vi "port_facade.vi"(0 "Data In":T4, 2 "Display State In":T2, 3 "Container State":T3) -> (6 "Data Out":T4, 7 "Display State Out":T2, 8 "Action":T1)   [LabVIEW 2024, in "portX.xctl"]
uses:
  Users/crogers/GitHub/ME121-25/LabVIEW/SerialVIs/subs/portX.xctl
  <userlib>/SerialVIs/subs/port_data.ctl
  <vilib>/_xctls/Container State.ctl
  <userlib>/SerialVIs/subs/port_state.ctl
  <vilib>/_xctls/Action.ctl
  <vilib>/_xctls/XControlSupport.lvlib
panel:
  in  "refresh":bool
  in  "Port":u16(ring)
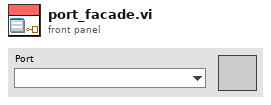
[diagram p1: front panel]
types:
  T1 = typedef "XControlSupport.lvlib/Action.ctl" = cluster{"Data Changed?":bool, "State Changed?":bool, "Action Name":string}
  T2 = typedef "portX.xctl/port_state.ctl" = cluster{"Numeric":dbl}
  T3 = typedef "XControlSupport.lvlib/Container State.ctl" = cluster{"Indicator?":bool, "Run Mode?":bool, " Refnum":refnum<vi>}
  T4 = typedef "portX.xctl/port_data.ctl" = refnum<visa-resource-name>
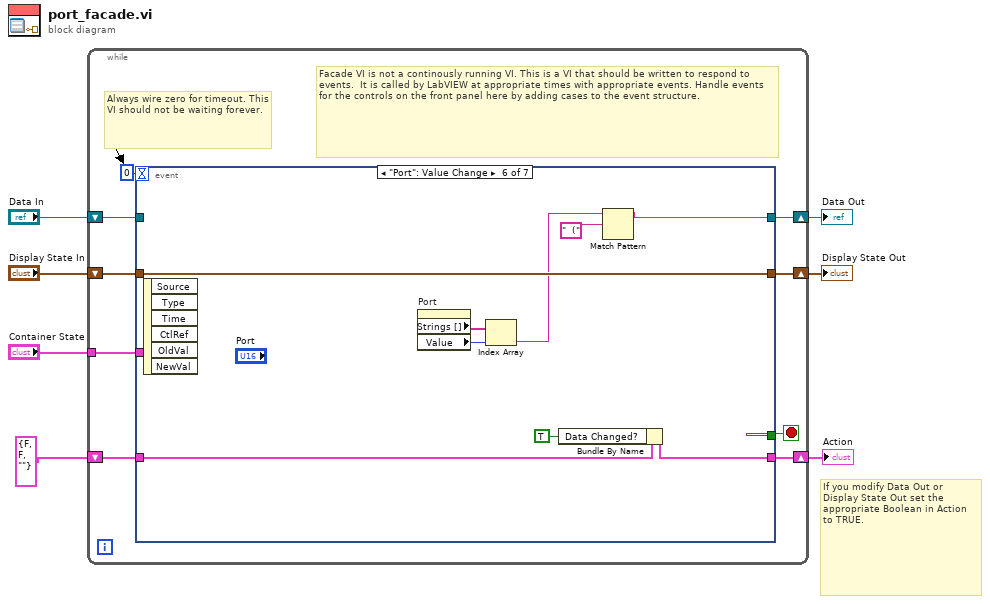
[diagram p0: block diagram]
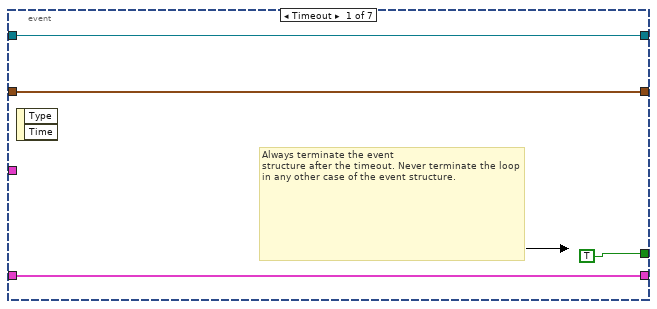
[diagram p2: hidden frame]
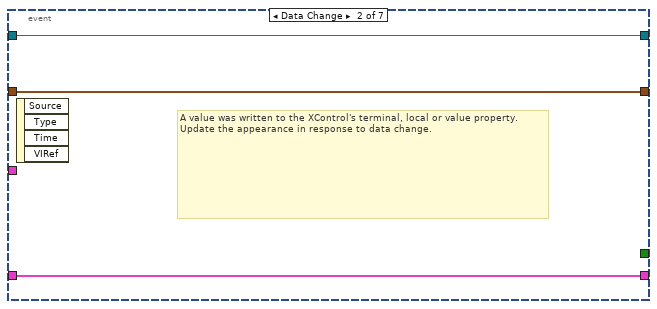
[diagram p3: hidden frame]
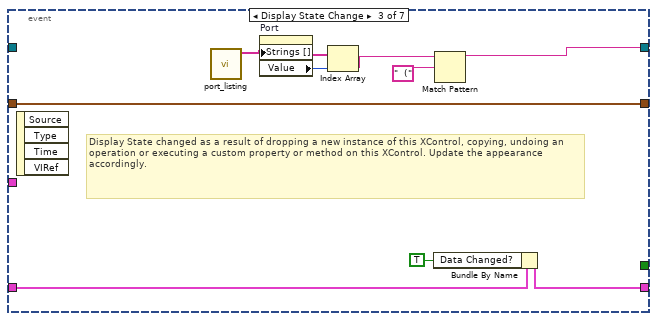
[diagram p4: hidden frame]
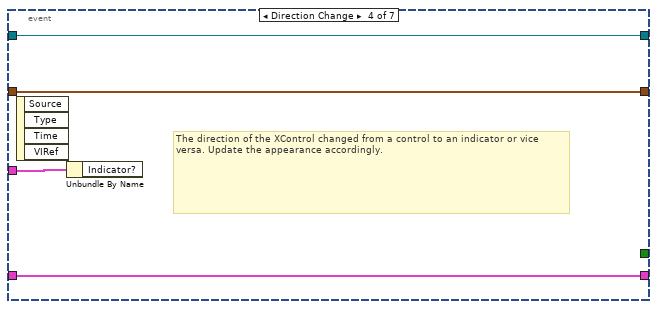
[diagram p5: hidden frame]
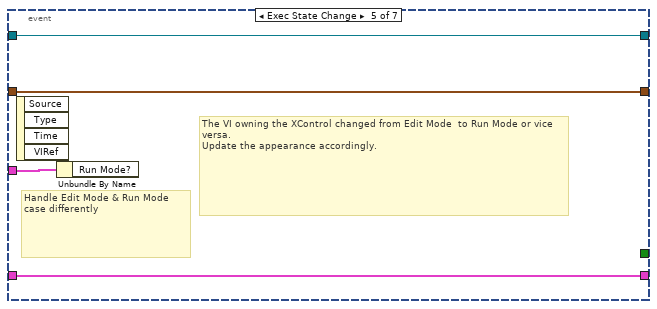
[diagram p6: hidden frame]
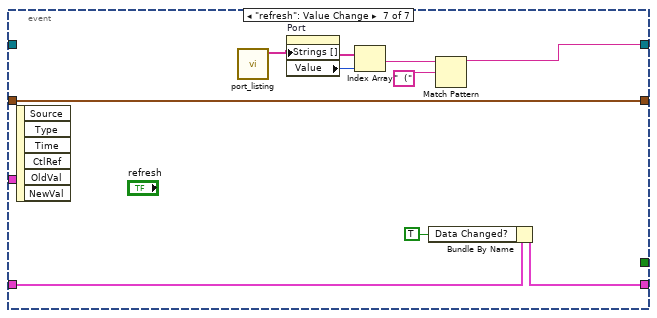
[diagram p7: hidden frame]
diagram:
  # "If you modify Data Out or\nDisplay State Out set the\nappropriate Boolean in Action\nto TRUE."
  n1 = while {
    shift-right: [w15] -> w4
    shift-left: "Display State In" -> [w16]
    tunnel: "Container State" -> [w12]
    shift-right: [w10] -> w7
    shift-left: "Data In" -> [w11]
    shift-right: [w8] -> w2
    shift-left: T1 {"Data Changed?"=FALSE, "State Changed?"=FALSE, "Action Name"=""} ("Action") -> [w9]
    stop <- w14 stop-if-true
    # "Facade VI is not a continously running VI. This is a VI that should be written to respond to events.  It is called by LabVIEW at appropriate times with appropriate events. Handle events for the controls on the front panel here by adding cases to the event structure."
    # "Always wire zero for timeout. This\nVI should not be waiting forever."
    n2 = event shown="[5] \"Port\": Value Change" {
      selector: _ -> [_ _ _ _ _ _ _]
      dyn-events: _ -> [_ _ _ _ _ _ _]
      timeout: 0 -> [_ _ _ _ _ _ _]
      tunnel: w16 -> [w18 w22 w32 w35 w39 w49 w58]
      tunnel: [w18 w22 w32 w35 w39 w49 w58] -> w15
      tunnel: [TRUE _ _ _ _ _ _] -> w14
      tunnel: w12 -> [_ _ _ w36 w40 _ _]
      tunnel: w11 -> [w17 w23 _ w34 w38 _ _]
      tunnel: [w17 w23 w24 w34 w38 w41 w50] -> w10
      tunnel: [w19 w21 w27 w33 w37 w44 w53] -> w8
      tunnel: w9 -> [w19 w21 w28 w33 w37 w45 w54]
      event Timeout {
        # "Always terminate the event\nstructure after the timeout. Never terminate the loop in any other case of the event structure."
        n3 = event-data() -> ()  [unwired: 1 in, 2 out]
      }
      event Data Change {
        # "A value was written to the XControl's terminal, local or value property.\nUpdate the appearance in response to data change."
        n4 = event-data() -> ()  [unwired: 1 in, 4 out]
      }
      event Display State Change {
        # "Display State changed as a result of dropping a new instance of this XControl, copying, undoing an operation or executing a custom property or method on this XControl. Update the appearance accordingly."
        n5 = event-data() -> ()  [unwired: 1 in, 4 out]
        n6 = call <userlib>:"port_listing.vi"() -> ("find list"=w30:string[])  [unwired: 9 in, 2 out]
        n7 = property on="Port" class="Ring (strict)"("Strings []"=w30) -> ("Value"=w31:u16)  [unwired: 2 in, 2 out]
        n8 = Index Array(array=w30, index=w31) -> (element=w25:string)
        n9 = Bundle By Name(cluster=w28, "Data Changed?"=TRUE) -> (w27:T1)
        n10 = Match Pattern(string=w25, regular expression="  (") -> (before substring=w24:string)  [unwired: 1 in, 3 out]
      }
      event Direction Change {
        # "The direction of the XControl changed from a control to an indicator or vice versa. Update the appearance accordingly."
        n11 = event-data() -> ()  [unwired: 1 in, 4 out]
        n12 = Unbundle By Name(w36) -> ()  [unwired: 1 out]
      }
      event Exec State Change {
        # "The VI owning the XControl changed from Edit Mode  to Run Mode or vice versa.\nUpdate the appearance accordingly."
        # "Handle Edit Mode & Run Mode\ncase differently"
        n13 = event-data() -> ()  [unwired: 1 in, 4 out]
        n14 = Unbundle By Name(w40) -> ()  [unwired: 1 out]
      }
      event "Port": Value Change {
        n15 = event-data() -> ()  [unwired: 1 in, 6 out]
        n16 = property on="Port" class="Ring (strict)"() -> ("Strings []"=w47:string[], "Value"=w48:u16)  [unwired: 2 in, 2 out]
        n17 = Index Array(array=w47, index=w48) -> (element=w42:string)
        n18 = Bundle By Name(cluster=w45, "Data Changed?"=TRUE) -> (w44:T1)
        n19 = Match Pattern(string=w42, regular expression="  (") -> (before substring=w41:string)  [unwired: 1 in, 3 out]
      }
      event "refresh": Value Change {
        n20 = event-data() -> ()  [unwired: 1 in, 6 out]
        n21 = call <userlib>:"port_listing.vi"() -> ("find list"=w56:string[])  [unwired: 9 in, 2 out]
        n22 = property on="Port" class="Ring (strict)"("Strings []"=w56) -> ("Value"=w57:u16)  [unwired: 2 in, 2 out]
        n23 = Index Array(array=w56, index=w57) -> (element=w52:string)
        n24 = Bundle By Name(cluster=w54, "Data Changed?"=TRUE) -> (w53:T1)
        n25 = Match Pattern(string=w52, regular expression="  (") -> (before substring=w50:string)  [unwired: 1 in, 3 out]
      }
    }
  }
  "Display State Out" <- w4
  "Data Out" <- w7
  "Action" <- w2
